vi "Contador1.vi"() -> ()   [LabVIEW 2020]
panel:
  out "Array":bool[](array[boolean])
  out "appended array":u64[](array[numeric])
  in  "stop":bool
  in  "Limite":u64
  out "Contador":dbl
  in  "Botón":bool
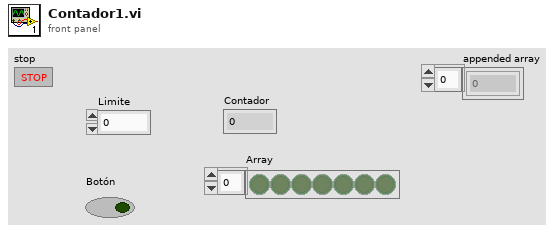
[diagram p1: front panel]
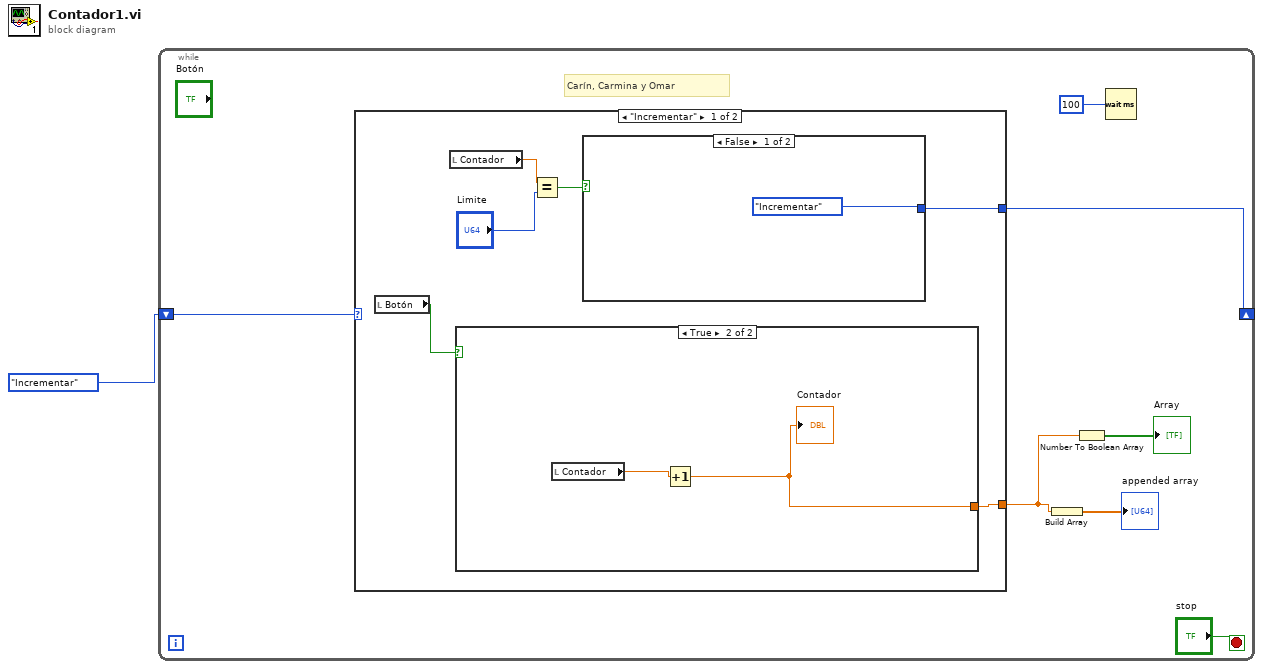
[diagram p0: block diagram]
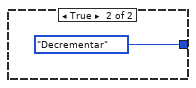
[diagram p2: hidden frame]
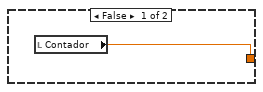
[diagram p3: hidden frame]
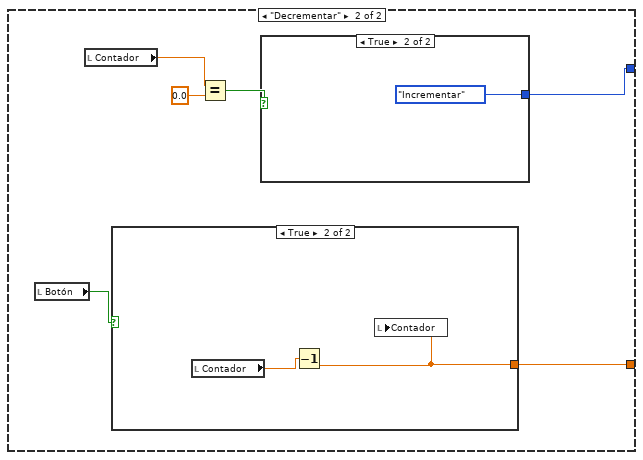
[diagram p4: hidden frame]
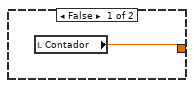
[diagram p5: hidden frame]
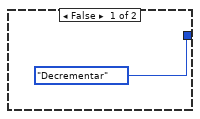
[diagram p6: hidden frame]
diagram:
  n1 = while {
    shift-right: [w5] -> _
    shift-left: enum16{"Decrementar", "Incrementar"}."Incrementar" -> [w8]
    stop <- "stop" stop-if-true
    # "Carín, Carmina y Omar"
    n2 = case shown="\"Incrementar\"" w8 {
      tunnel: [w10 w22] -> w3
      tunnel: [w9 w21] -> w5
      frame "Incrementar" {
        n3 = local read "Botón"() -> (w14:bool)
        n4 = local read "Contador"() -> (w12:dbl)
        n5 = case shown="True" w14 {
          tunnel: [w17 w18] -> w10
          frame False {
            n6 = local read "Contador"() -> (w17:dbl)
          }
          frame True {
            n7 = local read "Contador"() -> (w19:dbl)
            n8 = Increment(x=w19) -> (x+1=w18:dbl)
            "Contador" <- w18
          }
        }
        n9 = Equal?(x=w12, y="Limite") -> (x = y?=w13:bool)
        n10 = case shown="False" w13 {
          tunnel: [enum16{"Decrementar", "Incrementar"}."Incrementar" enum16{"Decrementar", "Incrementar"}."Decrementar"] -> w9
          frame False {
          }
          frame True {
          }
        }
      }
      frame "Decrementar" {
        n11 = local read "Botón"() -> (w23:bool)
        n12 = local read "Contador"() -> (w25:dbl)
        n13 = case shown="True" w23 {
          tunnel: [w26 w27] -> w22
          frame False {
            n14 = local read "Contador"() -> (w26:dbl)
          }
          frame True {
            n15 = local read "Contador"() -> (w28:dbl)
            n16 = Decrement(x=w28) -> (x-1=w27:dbl)
            n17 = local write "Contador"(w27) -> ()
          }
        }
        n18 = Equal?(x=w25, y=0.0) -> (x = y?=w24:bool)
        n19 = case shown="True" w24 {
          tunnel: [enum16{"Decrementar", "Incrementar"}."Decrementar" enum16{"Decrementar", "Incrementar"}."Incrementar"] -> w21
          frame False {
          }
          frame True {
          }
        }
      }
    }
    n20 = Build Array(w3) -> (→"appended array":dbl[])
    n21 = Number To Boolean Array(number=w3) -> (Boolean array=→"Array":bool[])
    n22 = Wait (ms)(milliseconds to wait=u32 100 ("millisecond timer value")) -> ()  [unwired: 1 out]
  }
